vi "Check Tag String.vi"(1 "String 2":string, 2 "String 1":string) -> (0 "equal":bool)   [LabVIEW 2021, in "PTU Files.lvlib"]
uses:
  PTU Files.lvlib
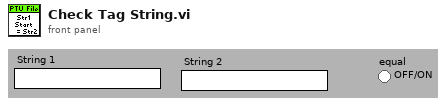
[diagram p1: front panel]
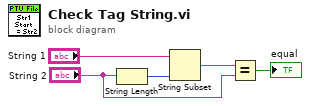
[diagram p0: block diagram]
diagram:
  n1 = String Length(string="String 2") -> (length=w5:i32)
  n2 = String Subset(string="String 1", length (rest)=w5) -> (substring=w3:string)  [unwired: 1 in]
  n3 = Equal?(x=w3, y="String 2") -> (x = y?=→"equal":bool)
